vi "Actor Core.vi"(8 "error in":errorcluster, 11 "Simple UI in":refnum<class "Simple UI.lvclass">) -> (0 "error out":errorcluster, 3 "Actor out":refnum<class "Actor.lvclass">)   [LabVIEW 2020, in "Simple UI.lvlib" / "Simple UI.lvclass"]
doc: "(<B>Filename</B>: Actor Framework.lvlib:Actor.lvclass:Actor Core.vi)\n\nReceives messages to the actor, reacts to them, and initiates any error handling that may shut the actor down.\n\nDescendant classes may override this VI to append parallel tasks for the actor to complete while it handles messages. Overrides use the Call Parent Class Method node."
uses:
  <vilib>/ActorFramework/Actor/Actor.lvclass
  <vilib>/ActorFramework/Actor/Actor.lvclass/Actor.ctl
  Simple UI.lvclass
  Base UI Actor/Base UI Actor/Base UI Actor.lvclass
  C:/Users/Ivan/Documents/AF Stop Helper Loop/Base UI Actor/Base UI Actor/Base UI Actor.lvclass
  C:/Program Files (x86)/National Instruments/LabVIEW 2020/vi.lib/ActorFramework/Actor/Actor.lvclass
  C:/Users/Ivan/Documents/AF Stop Helper Loop/Simple UI/Simple UI/Simple UI.lvclass
  <vilib>/ActorFramework/Stop Msg/Stop Msg.lvclass
panel:
  in  "_btn Stop":bool
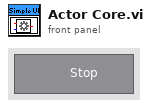
[diagram p1: front panel]
types:
  T1 = cluster{"accessors:StopHelperLoop Reg Ref":refnum<event-registration>}
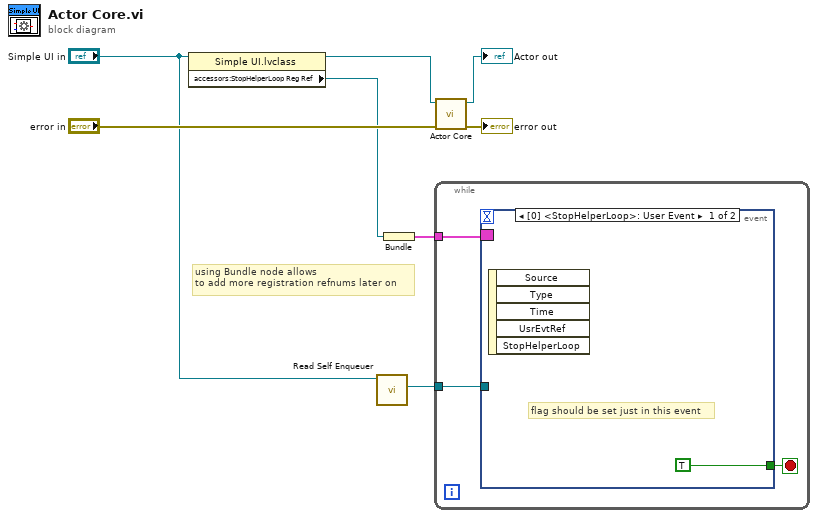
[diagram p0: block diagram]
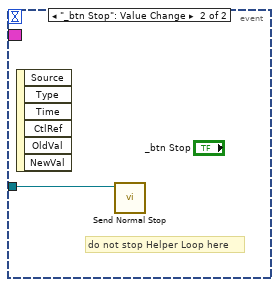
[diagram p2: hidden frame]
diagram:
  # "using Bundle node allows\nto add more registration refnums later on"
  n1 = property class="Simple UI.lvclass"(reference="Simple UI in") -> (reference out=w5:refnum<class "Simple UI.lvclass">, "accessors:StopHelperLoop Reg Ref"=w3:refnum<event-registration>)  [unwired: 1 in, 1 out]
  n2 = call <vilib>:"Read Self Enqueuer.vi"("Actor"="Simple UI in") -> ("Self Enqueuer"=w1:refnum<class "Message Enqueuer.lvclass">)  [unwired: 10 in]
  n3 = Bundle("accessors:StopHelperLoop Reg Ref"=w3) -> (w4:T1)  [unwired: 1 in]
  n4 = while {
    tunnel: w4 -> [w11]
    tunnel: w1 -> [w9]
    stop <- w10 stop-if-true
    n5 = event shown="[0] <StopHelperLoop>: User Event" {
      selector: w11 -> [_ _]
      dyn-events: _ -> [_ _]
      timeout: _ -> [_ _]
      tunnel: [TRUE _] -> w10
      tunnel: w9 -> [_ w13]
      event User Event {
        # "flag should be set just in this event"
        n6 = event-data() -> ()  [unwired: 1 in, 5 out]
      }
      event "_btn Stop": Value Change {
        # "do not stop Helper Loop here"
        n7 = event-data() -> ()  [unwired: 1 in, 6 out]
        n8 = call <vilib>:"Send Normal Stop.vi"("Message Enqueuer"=w13) -> ()  [unwired: 10 in, 1 out]
      }
    }
  }
  n9 = call-parent "Actor Core.vi"("error in"="error in", "Actor in"=w5) -> ("error out"=→"error out":errorcluster, "Actor out"=→"Actor out":refnum<class "Actor.lvclass">)  [unwired: 8 in]
